vi "Calibration_load_file.vi"() -> (1 "uABank1":dbl, 2 "USB_DEV":string, 3 "uABank0":dbl)   [LabVIEW 2015]
uses:
  <vilib>/Utility/config.llb/Read Key (Double).vi
  <vilib>/Utility/config.llb/Read Key (String).vi
  <vilib>/Utility/config.llb/NI_LVConfig.lvlib
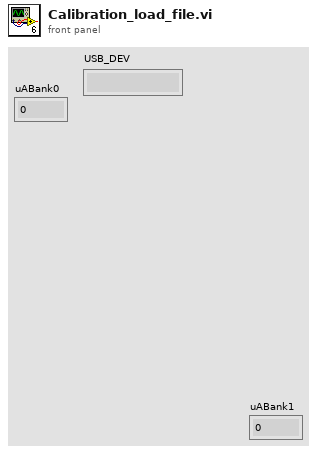
[diagram p1: front panel]
types:
  T1 = typedef "NI_LVConfig.lvlib/Config Data RefNum.ctl" = refnum<k1>
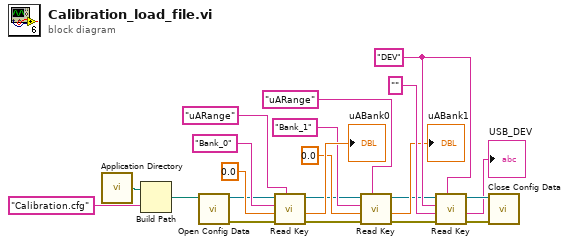
[diagram p0: block diagram]
diagram:
  w12 = "DEV" ("key")
  n1 = call <vilib>:"Application Directory.vi"() -> ("Application Directory"=w19:path)
  n2 = Build Path(base path=w19, name or relative path="Calibration.cfg") -> (appended path=w17:path)
  n3 = call <vilib>:"Open Config Data.vi"("configuration file path"=w17) -> ("error out"=w14:errorcluster, "refnum"=w16:T1)  [unwired: 8 in, 1 out]
  n4 = call-poly <vilib>:"Read Key.vi"("section"="uARange", "error in (no error)"=w14, "default value"=0.0, "key"="Bank_0", "refnum"=w16) -> ("error out"=w3:errorcluster, "value"=→"uABank0":dbl, "refnum out"=w4:T1)  [unwired: 3 in, 1 out]
  n5 = call-poly <vilib>:"Read Key.vi"("section"="uARange", "error in (no error)"=w3, "default value"=0.0, "key"="Bank_1", "refnum"=w4) -> ("error out"=w1:errorcluster, "value"=→"uABank1":dbl, "refnum out"=w2:T1)  [unwired: 3 in, 1 out]
  n6 = call-poly <vilib>:"Read Key.vi"("section"=w12, "error in (no error)"=w1, "default value"="", "key"=w12, "refnum"=w2) -> ("error out"=w9:errorcluster, "value"=→"USB_DEV":string, "refnum out"=w11:T1)  [unwired: 3 in, 1 out]
  n7 = call <vilib>:"Close Config Data.vi"("error in (no error)"=w9, "refnum"=w11) -> ()  [unwired: 8 in, 2 out]
